vi "Serial Loopback Async.vi"() -> ()   [LabVIEW 8.6]
uses:
  <libdir>/resource/objmgr/UeiDaq.rc
  <vilib>/UeiDaq/UeiDaqCreateSerialSession.vi
panel:
  out "String received":string
  out "Available bytes":i32
  out "Timestamp":u32
  in  "Watermark":i32
  in  "Mode":i32(ring) items=["RS-232", "RS-485 Half Duplex", "RS-485 Full Duplex"]
  out "String sent":string
  in  "Stop":bool
  in  "Number of characters to send\nat a time":i32
  in  "Bits per second":i32(ring) items=["110 bitsPerSecond", "300 bitsPerSecond", "600 bitsPerSecond", "1200 bitsPerSecond", "2400 bitsPerSecond", "4800 bitsPerSecond", "9600 bitsPerSecond", "14400 bitsPerSecond", "19200 bits PerSecond", "28800 bitsPerSecond", "38400 bitsPerSecond", "57600 bitsPerSecond", "115200 bitsPerSecond", "128000 bitsPerSecond", "256000 bitsPerSecond"]
  in  "Stop bits":i32(ring) items=["1 stop bit", "1.5 stop bits", "2 stop bits"]
  in  "Parity":i32(ring) items=["None", "Odd", "Even"]
  in  "Data bits":i32(ring) items=["5 data bits", "6 data bits", "7 data bits", "8 data bits"]
  out "device name":string
  in  "Resource":string
  # "Serial Loopback Async"
  # "1/ Set the resource name -->"
  # "Configure at least two ports in the resource string and connect the first two ports with a NULL-modem cable."
  # "2/ Configure Serial port -->"
  # "3/ Send/Receive -->"
  # "Device info"
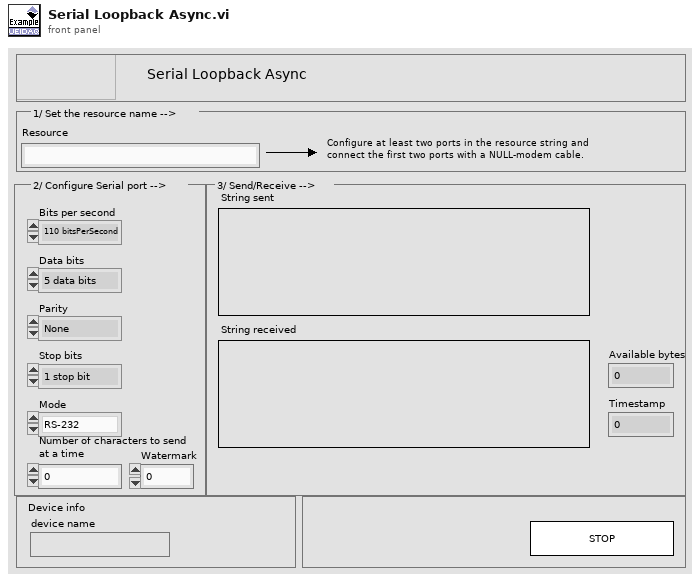
[diagram p1: front panel]
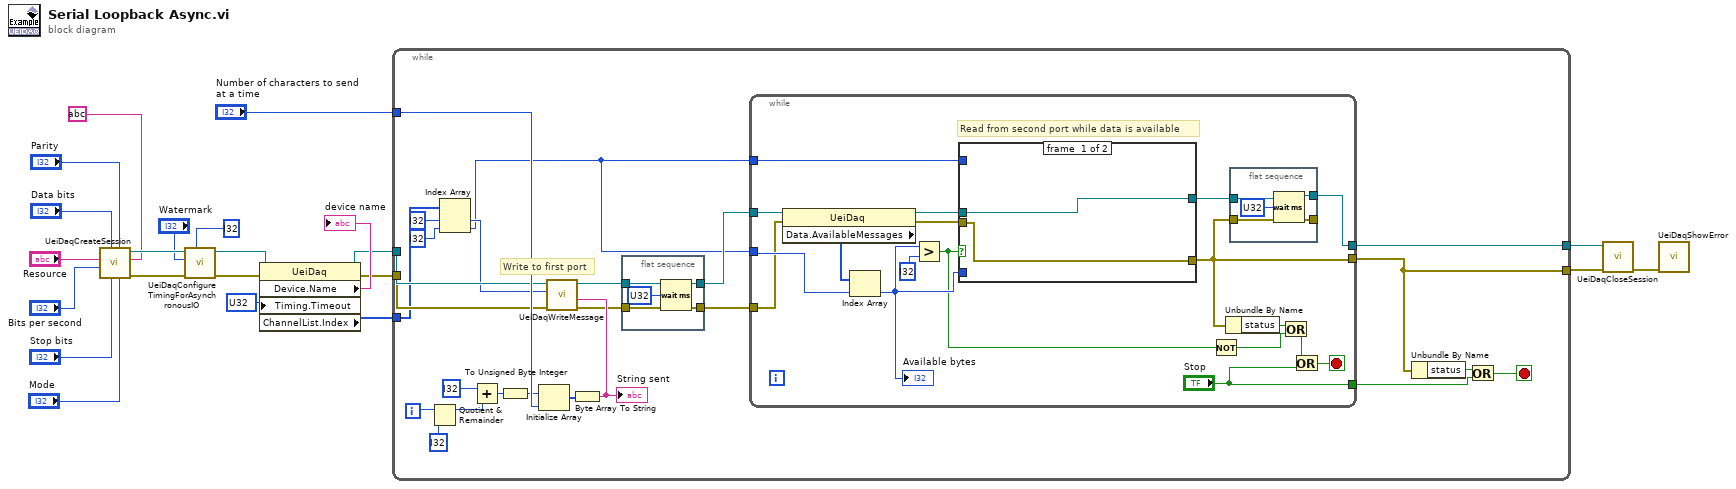
[diagram p0: block diagram]
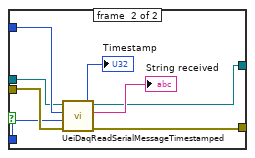
[diagram p2: hidden frame]
diagram:
  n1 = call-poly <vilib>:"UeiDaqCreateSession.vi"("Termination"=string ?, "Mode"="Mode", "Parity"="Parity", "Stop bits"="Stop bits", "Data bits"="Data bits", "Bits per second"="Bits per second", "Resource"="Resource") -> ("error out"=w19:errorcluster, "UeiDaq Refnum Out"=w20:refnum<k20>)  [unwired: 2 in, 1 out]
  n2 = call <vilib>:"UeiDaqConfigureTimingForAsynchronousIO.vi"("No activity timeout (us)"=i32 ?, "error in (no error)"=w19, "Watermark"="Watermark", "UeiDaq Refnum In"=w20) -> ("error out"=w16:errorcluster, "UeiDaq Refnum Out"=w17:refnum<k20>)  [unwired: 6 in]
  n3 = property class="UeiDaq"(reference=w17, error in=w16, "Timing.Timeout"=u32 ? ("Timing:Timeout")) -> (reference out=w9:refnum<k20>, error out=w8:errorcluster, "Device.Name"=→"device name":string, "ChannelList.Index"=w5:i32[])
  n4 = while {
    tunnel: w9 -> [w44]
    tunnel: w8 -> [w43]
    tunnel: [w37] -> w6
    tunnel: [w38] -> w7
    tunnel: "Number of characters to send\nat a time" -> [w45]
    tunnel: w5 -> [w41]
    i -> [w46]
    stop <- w42 stop-if-true
    # "Write to first port"
    n5 = Quotient & Remainder(x=w46, y=i32 ?) -> (x-y*floor(x/y)=w35:i32)  [unwired: 1 out]
    n6 = Index Array(array=w41, index #1=i32 ? ("index"), index #2=i32 ? ("index")) -> (element #1=w28:i32, element #2=w23:i32)
    n7 = Add(x=i32 ?, y=w35) -> (x+y=w33:i32)
    n8 = To Unsigned Byte Integer(number=w33) -> (unsigned 8bit integer=w32:u8)
    n9 = Initialize Array(w32, w45) -> (w31:u8[])
    n10 = Byte Array To String(unsigned byte array=w31) -> (string=w27:string)
    "String sent" <- w27
    n11 = call <vilib>:"UeiDaqWriteMessage.vi"("error in (no error)"=w43, "Message"=w27, "Port"=w28, "UeiDaq Refnum In"=w44) -> ("error out"=w26:errorcluster, "UeiDaq Refnum Out"=w25:refnum<k20>)  [unwired: 6 out]
    n12 = flat-sequence {
      tunnel: w26 -> [w81]
      tunnel: [w81] -> w39
      tunnel: w25 -> [w80]
      tunnel: [w80] -> w40
      frame #0 {
        n13 = Wait (ms)(milliseconds to wait=u32 ?) -> ()  [unwired: 1 out]
      }
    }
    n14 = while {
      tunnel: w23 -> [w64]
      tunnel: [w62] -> w38
      tunnel: [w53] -> w37
      tunnel: w39 -> [w61]
      tunnel: w40 -> [w60]
      tunnel: ["Stop"] -> w24
      tunnel: w23 -> [w55]
      stop <- w58 stop-if-true
      # "Read from second port while data is available"
      n15 = property class="UeiDaq"(reference=w60, error in=w61) -> (reference out=w54:refnum<k20>, error out=w56:errorcluster, "Data.AvailableMessages"=w65:i32[])
      n16 = Index Array(array=w65, index=w64) -> (element=w51:i32)
      "Available bytes" <- w51
      n17 = Greater?(x=w51, y=i32 ? ("milliseconds to wait")) -> (0:w49:bool)
      n18 = case shown="True" w49 {
        tunnel: w56 -> [w66 w75]
        tunnel: w51 -> [_ w74]
        tunnel: w55 -> [_ w73]
        tunnel: w54 -> [w67 w72]
        tunnel: [w66 w71] -> w53
        tunnel: [w67 w69] -> w52
        frame #0 {
        }
        frame #1 {
          n19 = call "UeiDaqReadSerialMessageTimestamped.vi"("error in (no error)"=w75, "byte count"=w74, "Port"=w73, "UeiDaq Refnum In"=w72) -> ("error out"=w71:errorcluster, "Message"=→"String received":string, "UeiDaq Refnum Out"=w69:refnum<k20>, "timestamp"=→"Timestamp":u32)  [unwired: 3 in, 1 out]
        }
      }
      n20 = Not(x=w49) -> (.not. x?=w48:bool)
      n21 = Unbundle By Name(w53) -> ("status"=w63:bool)
      n22 = flat-sequence {
        tunnel: [w78] -> _
        tunnel: w53 -> [w78]
        tunnel: w52 -> [w77]
        tunnel: [w77] -> w62
        frame #0 {
          n23 = Wait (ms)(milliseconds to wait=u32 ?) -> ()  [unwired: 1 out]
        }
      }
      n24 = Or(x=w63, y=w48) -> (x .or. y?=w59:bool)
      n25 = Or(x=w59, y="Stop") -> (x .or. y?=w58:bool)
    }
    n26 = Unbundle By Name(w37) -> ("status"=w47:bool)
    n27 = Or(x=w47, y=w24) -> (x .or. y?=w42:bool)
  }
  n28 = call <vilib>:"UeiDaqCloseSession.vi"("error in (no error)"=w6, "UeiDaq Refnum In"=w7) -> ("error out"=w21:errorcluster)  [unwired: 1 in, 8 out]
  n29 = call <vilib>:"UeiDaqShowError.vi"("error in (no error)"=w21) -> ()  [unwired: 2 in, 9 out]
